vi "Initialize Configuration Resource.vi"(8 "error in (no error)":errorcluster, 11 "database-configuration in":refnum<class "configuration-database.lvclass">) -> (0 "error out":errorcluster, 3 "database-configuration out":refnum<class "configuration-database.lvclass">)   [LabVIEW 2020, in "configuration-database.lvlib" / "configuration-database.lvclass"]
uses:
  configuration-database.lvclass
  configuration-database.lvclass/configuration-database.ctl
  9718e86e-9b64-4da2-852f-1426904affb1.vi
  <vilib>/Utility/error.llb/Error Cluster From Error Code.vi
  IConfigDBQueries/IConfigurationDatabaseQueries.lvclass
  externals/database-interface/IDatabase/IDatabase/IDatabase.lvclass
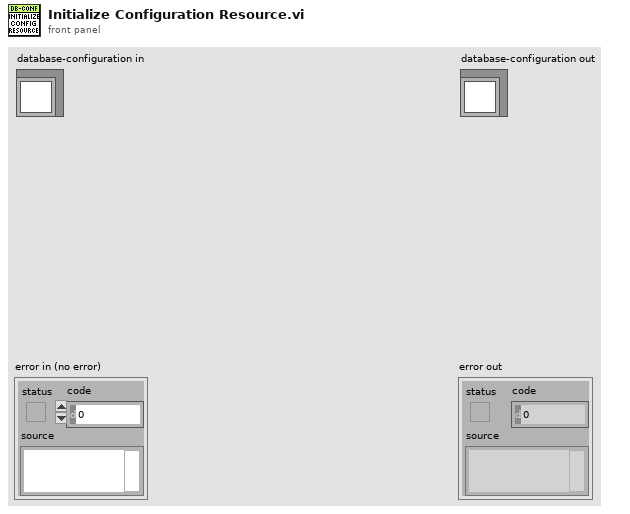
[diagram p1: front panel]
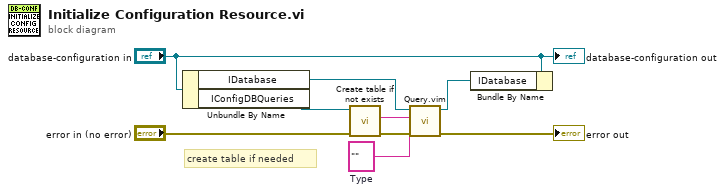
[diagram p0: block diagram]
diagram:
  w1 = ""  # Type
  # "create table if needed"
  n1 = Unbundle By Name("database-configuration in") -> ("IDatabase"=w5:refnum<class "IDatabase.lvclass">, "IConfigDBQueries"=w2:refnum<class "IConfigurationDatabaseQueries.lvclass">)
  n2 = call-dynamic "Create table if not exists.vi"("error in (no error)"="error in (no error)", "IConfigDBQueries in"=w2) -> ("error out"=w7:errorcluster, "Query out"=w3:string)  [unwired: 8 in]
  n3 = call "Query.vim"("error in (no error)"=w7, "Type and Default"=w1, "Query string"=w3, "IDatabase in"=w5) -> ("error out"=→"error out":errorcluster, "IDatabase out"=w4:refnum<class "IDatabase.lvclass">)  [unwired: 5 in, 1 out]
  n4 = Bundle By Name(cluster="database-configuration in", "IDatabase"=w4) -> ()  [unwired: 1 out]
  "database-configuration out" <- "database-configuration in"
